vi "prepAO_tt_v2.vi"() -> (0 "Terminal Name with Device Prefix":tag)   [LabVIEW 2015]
uses:
  <vilib>/DAQmx/write.llb/DAQmx Write (Analog 1D Wfm NChan NSamp).vi
  waveforms/usedAOindepofwf.vi
  Misc/add channel to active arrayv2.vi
  Objects/configuration.vi
  Objects/waveformsAObuffer.vi
  <vilib>/DAQmx/create/channels.llb/DAQmx Create Channel (AO-Voltage-Basic).vi
  <vilib>/DAQmx/configure/timing.llb/DAQmx Timing (Sample Clock).vi
  <vilib>/DAQmx/configure/trigger.llb/DAQmx Start Trigger (Digital Edge).vi
  <vilib>/DAQmx/miscellaneous.llb/DAQmx Fill In Error Info.vi
  <resource>/objmgr/daqmx.rc
panel:
  in  "error in 3":errorcluster caption="error in"
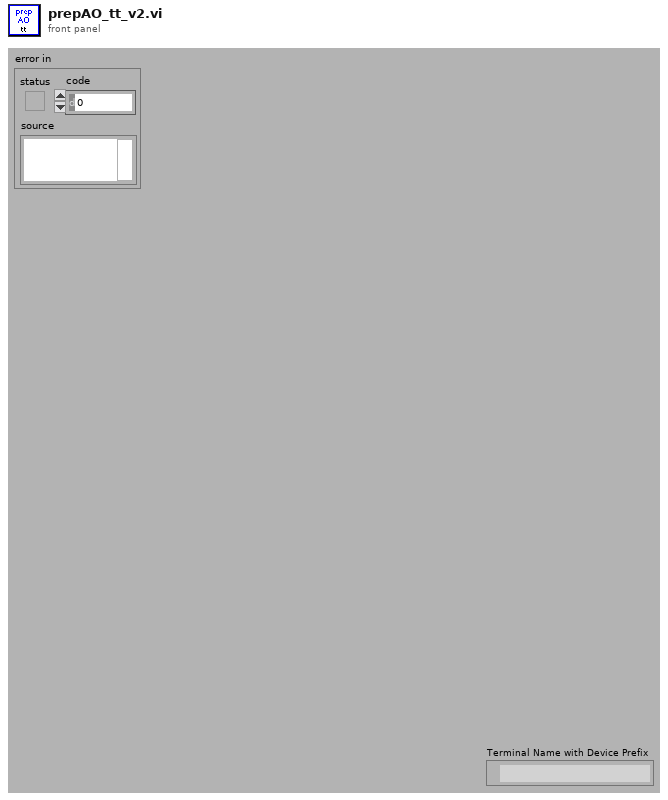
[diagram p1: front panel]
types:
  T1 = cluster{"presorted indices":i32[], "AOchans in this device":tag[], "usedAO sorted":i32[]}[]
  T2 = cluster{"Terminal Name with Device Prefix":tag, "RefClk.Src":tag, "RefClk.Rate":dbl}
  T3 = typedef "LVRectTypeDef.ctl" = cluster{"Left":i16, "Top":i16, "Right":i16, "Bottom":i16}
  T4 = cluster{"Xpixels":i32, "Vxminref":dbl, "Vxmaxref":dbl, "P":dbl, "Ypixels":i32, "Vyminref":dbl, "Vymaxref":dbl, "srate":sgl, "sAOxy":i32, "timeout":dbl, "type":string, "date":string, "time":string, "Colormap":u16, "Drawing Mode":u16, "Scanning Mode":u16, "square pixels":bool, "square matrix":bool, "Xpixels Img":i32, "Vx-min Img":dbl, "VX-max Img":dbl, "Ypixels Img":i32, "Vy-min Img":dbl, "Vy-max Img ":dbl, "Angle Img":dbl, "autoshutter":bool, "finite":bool, "cont":bool, "wavdet":bool, "measpoints":i32, "avpp":i32, "bufferAO":i32, "bufferAI":i32, "starttick":u32, "waveform":path, "Vx-ref":dbl, "Vy-ref":dbl, "refreshrate":dbl, "refreshbuffer":i32, "tt_cycles":i32, "motorref":refnum<k7>, "mirrorswitch":refnum<k7>, "sample mode":i32, "maxbufferAI":i32, "srateAODO":sgl, "bin":sgl, "Pel":sgl, "Angle draw":dbl, "srate Img":sgl, "ROIimg_plotbounds":T3, "auto OD":bool, "ODfilt":u16, "aAI":i32[], "aCI":i32[], "aAO":u32[], "aDO":u32[], "refwfsize":dbl, "Lifetime":bool, "Vz-Img":dbl, "Vz-ref":dbl, "Vz-reset":dbl, "AIoverride":bool}
  T5 = cluster{"AO":refnum<k21>[], "E_AO":errorcluster[]}
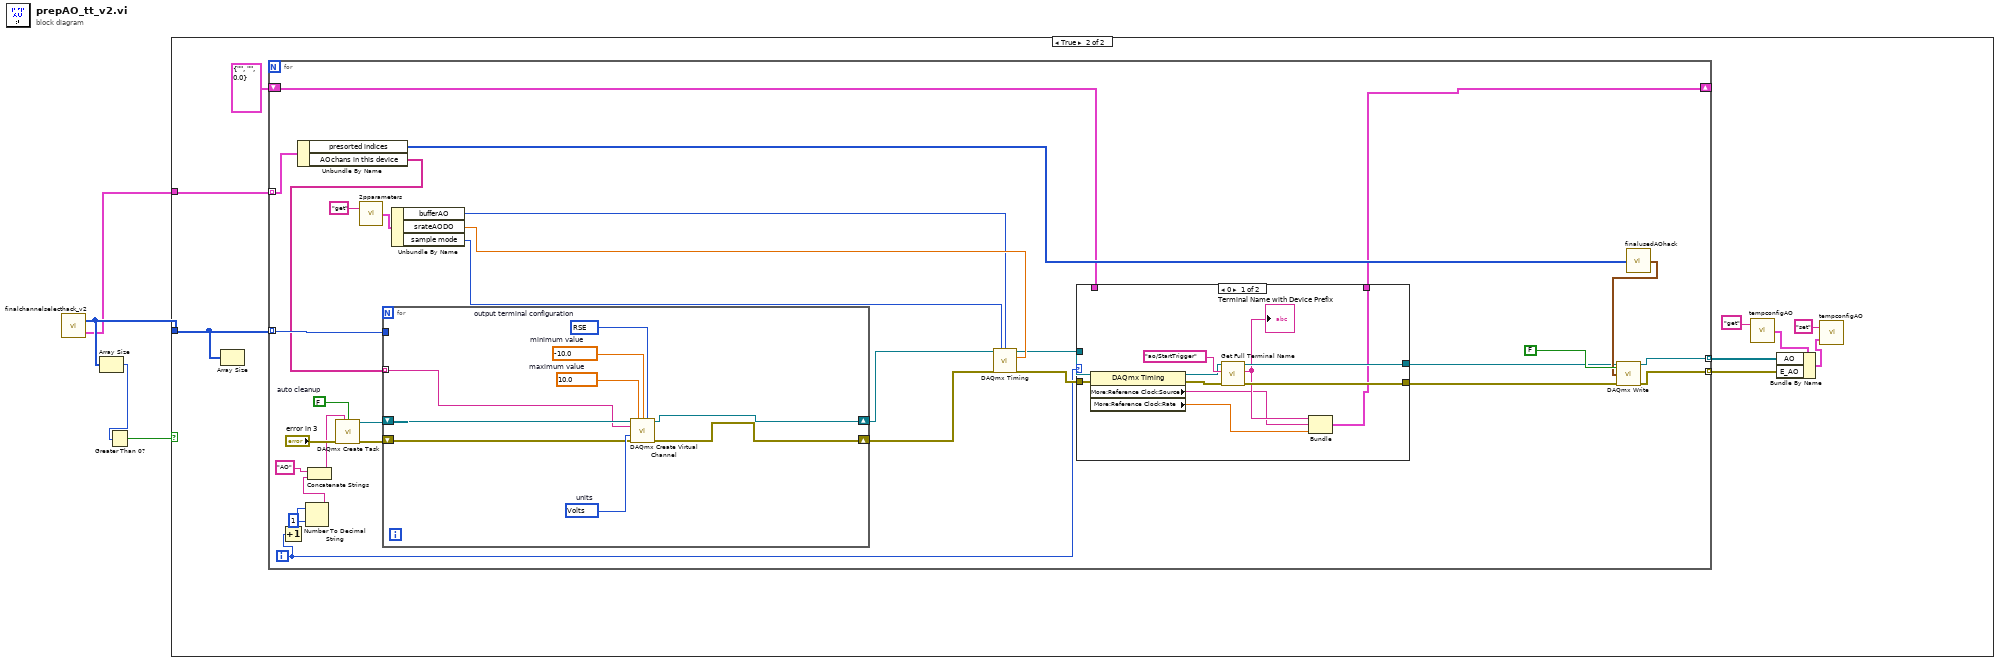
[diagram p0: block diagram]
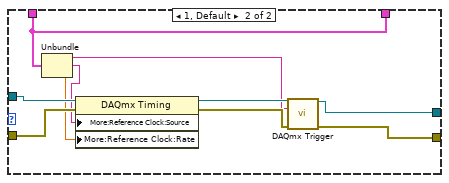
[diagram p3: hidden frame]
diagram:
  n1 = call "finalchannelselecthack_v2.vi"() -> ("devices"=w2:u32[], "Device chans"=w1:T1)  [unwired: 1 in]
  n2 = Array Size(array=w2) -> (size(s)=w3:i32)
  n3 = Greater Than 0?(x=w3) -> (x > 0?=w4:bool)
  n4 = case shown="True" w4 {
    tunnel: w2 -> [_ w5]
    tunnel: w1 -> [_ w13]
    frame False {
    }
    frame True {
      n5 = Array Size(array=w5) -> ()  [unwired: 1 out]
      n6 = for {
        tunnel: w5 -> [w40] mode=indexing
        tunnel: w13 -> [w30] mode=indexing
        tunnel: [w20] -> w8 mode=indexing
        tunnel: [w19] -> w7 mode=indexing
        shift-right: [w15] -> _
        shift-left: T2 {"Terminal Name with Device Prefix"="", "RefClk.Src"="", "RefClk.Rate"=0.0} -> [w16]
        i -> [w14]
        w42 = FALSE  # auto cleanup
        n7 = Increment(x=w14) -> (x+1=w27:i32)
        n8 = Unbundle By Name(w30) -> ("presorted indices"=w23:i32[], "AOchans in this device"=w29:tag[])
        n9 = Number To Decimal String(number=w27, width (-)=i16 1) -> (decimal integer string=w26:string)
        n10 = Concatenate Strings("AO" ("new task name"), w26) -> (w24:string)
        n11 = call <vilib>:"DAQmx Create Task.vi"("new task name"=w24, "auto cleanup"=w42, "error in"="error in 3") -> ("task out"=w43:refnum<k21>, "error out"=w44:errorcluster)  [unwired: 11 in]
        n12 = call "2pparameters.vi"("command"="get") -> ("params out"=w35:T4)  [unwired: 1 in]
        n13 = for {
          shift-right: [w68] -> w39
          shift-left: w43 -> [w70]
          shift-right: [w67] -> w38
          shift-left: w44 -> [w69]
          tunnel: w40 -> [_]
          tunnel: w29 -> [w66] mode=indexing
          w74 = 10083 items=["Default"=-1, "RSE"=10083, "Differential"=10106, "Pseudodifferential"=12529]  # output terminal configuration
          w73 = 10348 items=["Volts"=10348, "From Custom Scale"=10065]  # units
          w72 = -10.0  # minimum value
          w71 = 10.0  # maximum value
          n14 = call-poly <vilib>:"DAQmx Create Virtual Channel.vi"("task in"=w70, "maximum value"=w71, "minimum value"=w72, "output terminal configuration"=w74, "physical channels"=w66, "units"=w73, "error in"=w69) -> ("task out"=w68:refnum<k21>, "error out"=w67:errorcluster)  [unwired: 7 in]
        }
        n15 = Unbundle By Name(w35) -> ("bufferAO"=w32:i32, "srateAODO"=w33:sgl, "sample mode"=w34:i32)
        n16 = call-poly <vilib>:"DAQmx Timing.vi"("task/channels in"=w39, "sample mode"=w34, "samples per channel"=w32, "rate"=w33, "error in"=w38) -> ("task out"=w17:refnum<k21>, "error out"=w18:errorcluster)  [unwired: 2 in, 7 out]
        n17 = case shown="0" w14 {
          tunnel: [w54 w61] -> w22
          tunnel: [w53 w60] -> w21
          tunnel: w18 -> [w52 w64]
          tunnel: w17 -> [w51 w65]
          tunnel: w16 -> [_ w59]
          tunnel: [w45 w59] -> w15
          frame 0 {
            n18 = property class="DAQmx Timing"(reference=w51, error in=w52) -> (reference out=w50:refnum<k21>, error out=w49:errorcluster, "More:Reference Clock:Source"=w46:tag, "More:Reference Clock:Rate"=w47:dbl)
            n19 = call "Get Full Terminal Name.vi"("error in"=w49, "Local Terminal Name"="ao/StartTrigger", "task/channels in"=w50) -> ("error out"=w53:errorcluster, "Terminal Name with Device Prefix"=w48:tag, "task out"=w54:refnum<k21>)  [unwired: 6 in]
            "Terminal Name with Device Prefix" <- w48
            n20 = Bundle("Terminal Name with Device Prefix"=w48, "RefClk.Src"=w46, "RefClk.Rate"=w47) -> (w45:T2)  [unwired: 1 in]
          }
          frame 1, Default {
            n21 = Unbundle(w59) -> ("Terminal Name with Device Prefix"=w58:tag, "RefClk.Src"=w57:tag, "RefClk.Rate"=w56:dbl)
            n22 = property class="DAQmx Timing"(reference=w65, error in=w64, "More:Reference Clock:Source"=w57, "More:Reference Clock:Rate"=w56) -> (reference out=w63:refnum<k21>, error out=w62:errorcluster)
            n23 = call-poly <vilib>:"DAQmx Trigger.vi"("task/channels in"=w63, "source"=w58, "error in"=w62) -> ("task out"=w61:refnum<k21>, "error out"=w60:errorcluster)  [unwired: 11 in]
          }
        }
        n24 = call "finalusedAOhack.vi"("presorted indices"=w23) -> ("AO wf out"=w31:waveform(dbl)[])
        n25 = call-poly <vilib>:"DAQmx Write.vi"("task/channels in"=w22, "auto start"=FALSE, "data"=w31, "error in"=w21) -> ("task out"=w20:refnum<k21>, "error out"=w19:errorcluster)  [unwired: 9 in, 1 out]
      }
      n26 = call "tempconfigAO.vi"("command"="get") -> ("Temp Config out"=w11:T5)  [unwired: 1 in]
      n27 = Bundle By Name(cluster=w11, "AO"=w8, "E_AO"=w7) -> (w12:T5)
      n28 = call "tempconfigAO.vi"("Temp Config in"=w12, "command"="set") -> ()  [unwired: 1 out]
    }
  }
